vi "FpgaLink_Initialize.vi"(8 "error in (no error)":errorcluster) -> (0 "error out":errorcluster)   [LabVIEW 2011]
doc: "Initialise the library."
uses:
  libfpgalink.dll
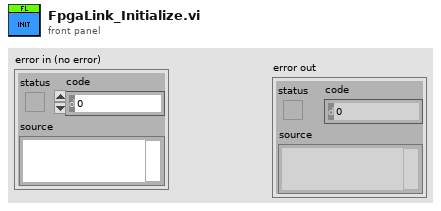
[diagram p1: front panel]
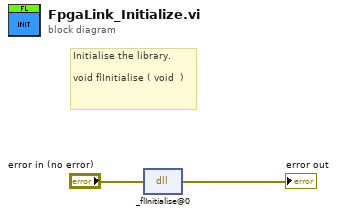
[diagram p0: block diagram]
diagram:
  # "Initialise the library.\n\nvoid flInitialise\t(\tvoid\t\t)"
  n1 = dll-call lib="libfpgalink.dll" fn="_flInitialise@0"(error in="error in (no error)") -> (error out=→"error out":errorcluster)  [unwired: 3 in, 1 out]
